vi "DI Reliability Test.vi"() -> ()   [LabVIEW 2015]
uses:
  <vilib>/Platform/TimedLoop/XDataNode/timing_clust.ctl
  <vilib>/Platform/TimedLoop/XDataNode/nitl_modes.ctl
  <vilib>/Platform/TimedLoop/XDataNode/wakeup.ctl
  <vilib>/DAQmx/read.llb/DAQmx Read (Digital Bool 1Line 1Point).vi
  <vilib>/DAQmx/create/channels.llb/DAQmx Create Channel (DI-Digital Input).vi
  <vilib>/DAQmx/miscellaneous.llb/DAQmx Fill In Error Info.vi
  <vilib>/platform/TimedLoop/XDataNode/XDataNode.xnode
  <vilib>/Platform/TimedLoop/XDataNode/XDNodeRunTimeDep.lvlib
  <vilib>/DAQmx/create/channels.llb/DAQmx Create Channel (AO-Voltage-Basic).vi
  <vilib>/DAQmx/configure/timing.llb/DAQmx Timing (Sample Clock).vi
  <resource>/objmgr/daqmx.rc
  <vilib>/DAQmx/write.llb/DAQmx Write (Analog 1D DBL 1Chan NSamp).vi
  <vilib>/Analysis/NI_AALBase.lvlib
panel:
  out "SpaceAvail":u32
  in  "stop 2":bool
  out "Waveform Graph":i64[](graph)
  in  "lines":tag
  out "error out":errorcluster
  in  "stop":bool
  out "Triggers":i32
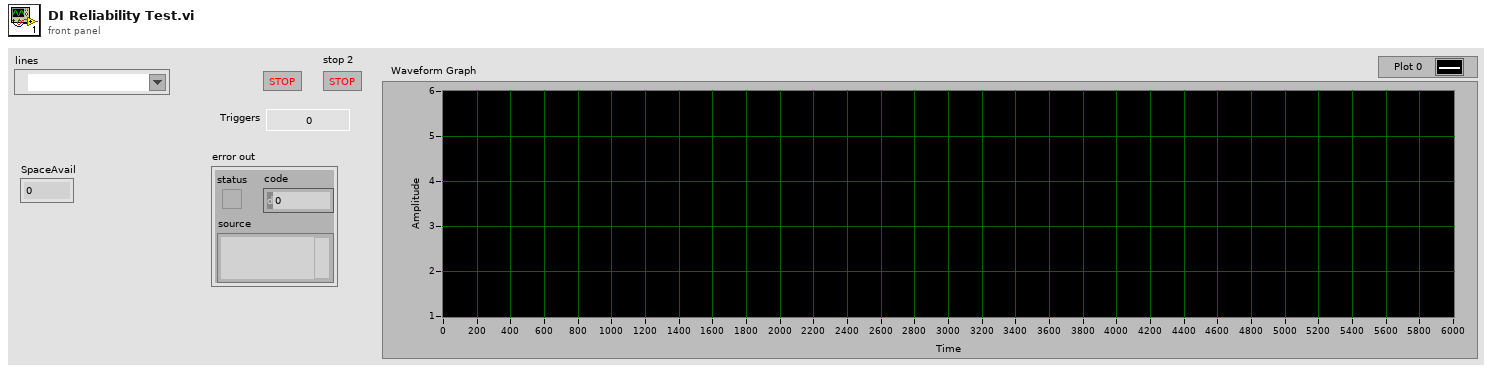
[diagram p1: front panel]
types:
  T1 = typedef "XDNodeRunTimeDep.lvlib/timing_clust.ctl" = cluster{"Expected End [f-1]":u64, "Actual End [f-1]":u64, "Finished Late? [f-1]":bool, "Expected End [i-1]":u64, "Actual End [i-1]":u64, "Finished Late? [i-1]":bool, "Expected Start [i]":u64, "Actual Start [i]":u64, "Expected Start [f]":u64, "Actual Start [f]":u64, "Source Name":string, "Structure Name":string, "Period":i64, "Deadline":i64, "Offset":i64, "Start":i64, "Priority":i32, "Timeout":i32, "Mode":T2, "Wakeup Reason":T3, "Error":errorcluster, "Source Type":string, "Secondary Source Type":string, "Global End Time":u64, "Global Start Time":u64, "Frame Duration":u64, "Iteration Duration":u64, "Assigned CPU":i32, "I/O Scan Engine Mode":u32}
  T2 = typedef "XDNodeRunTimeDep.lvlib/nitl_modes.ctl" = enum32{"No Change", "Process missed periods, maintain original phase", "Discard missed periods, maintain original phase", "Process missed periods, ignore original phase", "Discard missed periods, ignore original phase"}
  T3 = typedef "XDNodeRunTimeDep.lvlib/wakeup.ctl" = enum32{"Normal", "Aborted", "Asynchronous wakeup", "Timing source error", "Timed loop error", "Timeout"}
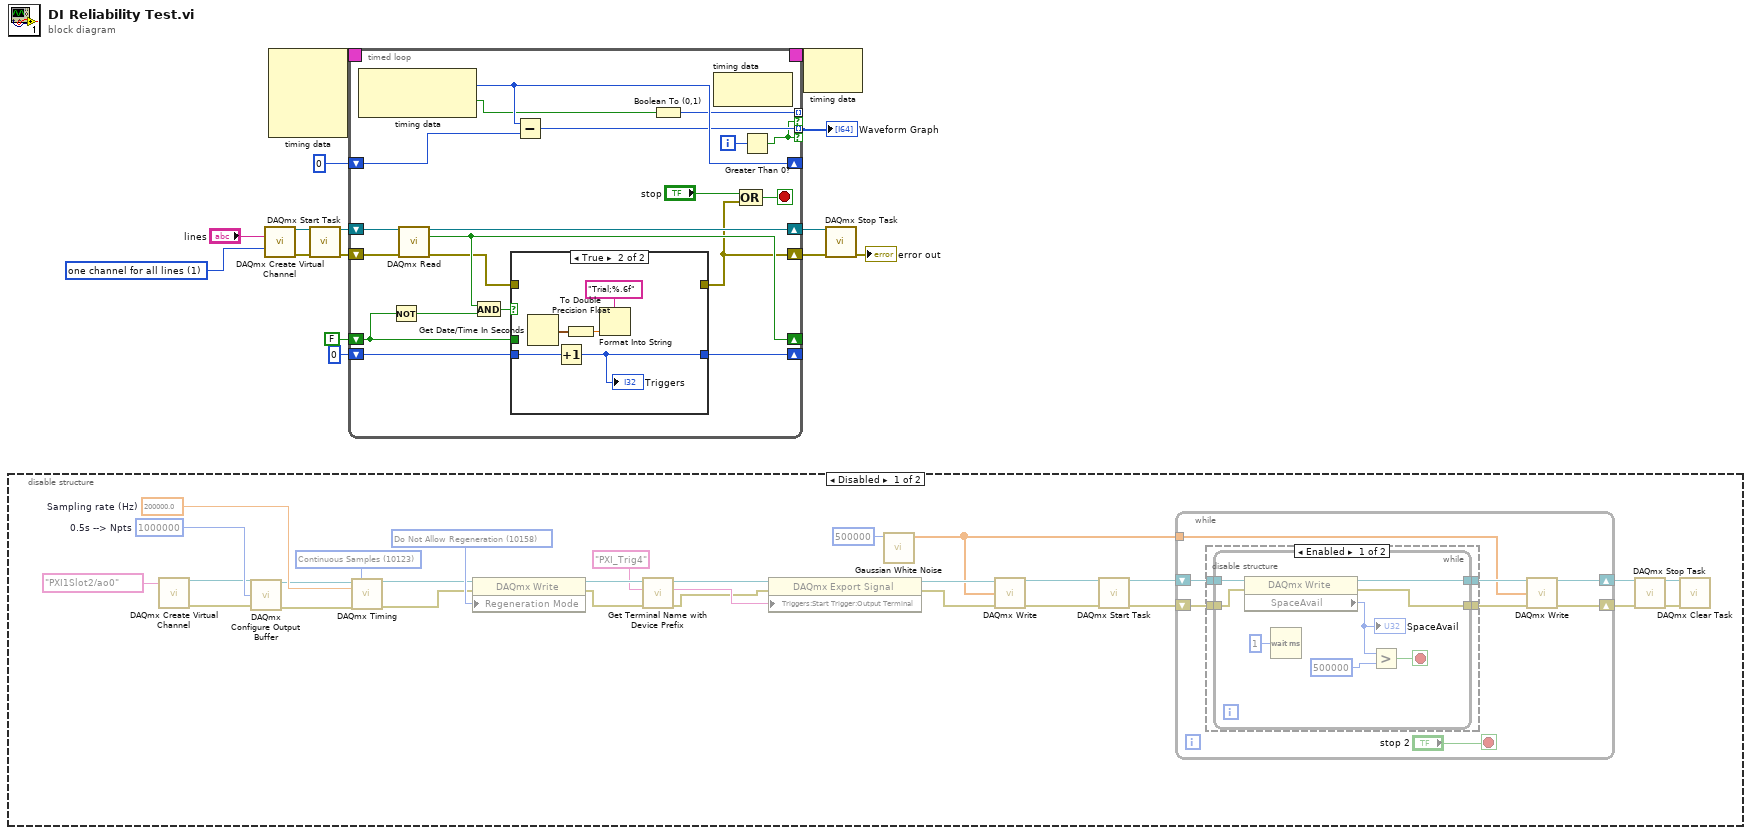
[diagram p0: block diagram]
diagram:
  w11 = 1 items=["one channel for each line", "one channel for all lines"] ("line grouping")
  n1 = disable-structure shown="Disabled" {
    frame Disabled {
      w41 = 200000.0  # Sampling rate (Hz)
      w43 = 1000000  # 0.5s --> Npts
      w25 = 10123 items=["Finite Samples"=10178, "Continuous Samples"=10123, "Hardware Timed Single Point"=12522] ("sample mode")
      w21 = 10158 items=["Allow Regeneration"=10097, "Do Not Allow Regeneration"=10158] ("RegenMode")
      n2 = call-poly <vilib>:"DAQmx Create Virtual Channel.vi"("physical channels"=tag "PXI1Slot2/ao0") -> ("task out"=w17:refnum<k21>, "error out"=w22:errorcluster)  [unwired: 13 in]
      n3 = call <vilib>:"DAQmx Configure Output Buffer.vi"("task/channels in"=w17, "buffer size (in samples per channel)"=w43, "error in"=w22) -> ("task out"=w18:refnum<k21>, "error out"=w23:errorcluster)  [unwired: 11 in]
      n4 = call-poly <vilib>:"DAQmx Timing.vi"("task/channels in"=w18, "sample mode"=w25, "rate"=w41, "error in"=w23) -> ("task out"=w20:refnum<k21>, "error out"=w19:errorcluster)  [unwired: 10 in]
      n5 = property class="DAQmx Write"(reference=w20, error in=w19, "Regeneration Mode"=w21) -> (reference out=w29:refnum<k21>, error out=w30:errorcluster)
      n6 = call "Get Terminal Name with Device Prefix.vi"("error in (no error)"=w30, "Local Terminal Name"="PXI_Trig4", "task/channels in"=w29) -> ("error out"=w27:errorcluster, "Terminal Name with Device Prefix"=w44:tag, "task out"=w28:refnum<k21>)  [unwired: 6 in]
      n7 = property class="DAQmx Export Signal"(reference=w28, error in=w27, "Triggers:Start Trigger:Output Terminal"=w44) -> (reference out=w37:refnum<k21>, error out=w39:errorcluster)
      n8 = call <vilib>:"Gaussian White Noise.vi"("samples"=500000) -> ("Gaussian noise pattern"=w16:dbl[])  [unwired: 9 in, 1 out]
      n9 = call-poly <vilib>:"DAQmx Write.vi"("task/channels in"=w37, "data"=w16, "error in"=w39) -> ("task out"=w38:refnum<k21>, "error out"=w40:errorcluster)  [unwired: 10 in, 1 out]
      n10 = call <vilib>:"DAQmx Start Task.vi"("task/channels in"=w38, "error in"=w40) -> ("task out"=w32:refnum<k21>, "error out"=w31:errorcluster)  [unwired: 12 in]
      n11 = while {
        shift-right: [w48] -> w33
        shift-left: w32 -> [w52]
        shift-right: [w46] -> w34
        shift-left: w31 -> [w51]
        tunnel: w16 -> [w45]
        stop <- "stop 2" stop-if-true
        n12 = disable-structure shown="Enabled" {
          disable-tunnel: w52 -> [w56 w66]
          disable-tunnel: w51 -> [w55 w65]
          disable-tunnel: [w54 w66] -> w49
          disable-tunnel: [w53 w65] -> w47
          frame Enabled {
            n13 = while {
              tunnel: w55 -> [w62]
              tunnel: w56 -> [w63]
              tunnel: [w61] -> w54
              tunnel: [w60] -> w53
              stop <- w58 stop-if-true
              n14 = property class="DAQmx Write"(reference=w63, error in=w62) -> (reference out=w61:refnum<k21>, error out=w60:errorcluster, "SpaceAvail"=w59:u32)
              "SpaceAvail" <- w59
              n15 = Wait (ms)(milliseconds to wait=u32 1) -> ()  [unwired: 1 out]
              n16 = Greater?(x=w59, y=500000 ("samples")) -> (0:w58:bool)
            }
          }
          frame Disabled {
          }
        }
        n17 = call-poly <vilib>:"DAQmx Write.vi"("task/channels in"=w49, "data"=w45, "error in"=w47) -> ("task out"=w48:refnum<k21>, "error out"=w46:errorcluster)  [unwired: 10 in, 1 out]
      }
      n18 = call <vilib>:"DAQmx Stop Task.vi"("task/channels in"=w33, "error in"=w34) -> ("task out"=w35:refnum<k21>, "error out"=w36:errorcluster)  [unwired: 12 in]
      n19 = call <vilib>:"DAQmx Clear Task.vi"("task in"=w35, "error in"=w36) -> ()  [unwired: 13 in, 1 out]
    }
    frame Enabled {
    }
  }
  n20 = call-poly <vilib>:"DAQmx Create Virtual Channel.vi"("lines"="lines", "line grouping"=w11) -> ("task out"=w6:refnum<k21>, "error out"=w5:errorcluster)  [unwired: 12 in]
  n21 = node-c288() -> (w15:T1)  [unwired: 4 in]
  n22 = call <vilib>:"DAQmx Start Task.vi"("task/channels in"=w6, "error in"=w5) -> ("task out"=w8:refnum<k21>, "error out"=w7:errorcluster)  [unwired: 12 in]
  n23 = timed-loop {
    shift-right: [w79] -> _
    shift-left: FALSE -> [w81]
    shift-right: [w77] -> _
    shift-left: 0 -> [w78]
    timing: w15 -> [_]
    timing-out: [_] -> w14
    shift-right: [w83] -> w10
    shift-left: w8 -> [w85]
    shift-right: [w74] -> w9
    shift-left: w7 -> [w84]
    shift-right: [w73] -> _
    shift-left: 0 -> [w72]
    tunnel: [w71] -> w1 mode=indexing if=w67
    tunnel: [w68] -> _ mode=indexing if=w67
    i -> [w70]
    stop <- w86 stop-if-true
    n24 = node-c288() -> (w73:i64, w69:bool)  [unwired: 1 in]
    n25 = Not(x=w81) -> (.not. x?=w80:bool)
    n26 = call-poly <vilib>:"DAQmx Read.vi"("task/channels in"=w85, "error in"=w84) -> ("task out"=w83:refnum<k21>, "data"=w79:bool, "error out"=w76:errorcluster)  [unwired: 11 in]
    n27 = And(x=w79, y=w80) -> (x .and. y?=w82:bool)
    n28 = case shown="True" w82 {
      tunnel: [w91 _] -> w74
      tunnel: w81 -> [_ _]
      tunnel: w78 -> [w92 w94]
      tunnel: [w92 w93] -> w77
      tunnel: w76 -> [w91 _]
      frame False {
      }
      frame True {
        n29 = Get Date/Time In Seconds() -> (seconds since 1Jan1904=w96:timestamp)
        n30 = Increment(x=w94) -> (x+1=w93:i32)
        "Triggers" <- w93
        n31 = To Double Precision Float(number=w96) -> (double precision float=w95:dbl)
        n32 = Format Into String(format string="Trial;%.6f", w95) -> ()  [unwired: 2 in, 2 out]
      }
    }
    n33 = Subtract(x=w73, y=w72) -> (x-y=w71:i64)
    n34 = Boolean To (0,1)(Boolean=w69) -> (0, 1=w68:i16)
    n35 = node-c288() -> ()  [unwired: 1 in, 1 out]
    n36 = Compound Arithmetic op=OR("stop", w74) -> (w86:bool)
    n37 = Greater Than 0?(x=w70) -> (x > 0?=w67:bool)
  }
  "Waveform Graph" <- w1
  n38 = node-c288(w14) -> ()  [unwired: 1 out]
  n39 = call <vilib>:"DAQmx Stop Task.vi"("task/channels in"=w10, "error in"=w9) -> ("error out"=→"error out":errorcluster)  [unwired: 12 in, 1 out]
